vi "SetStringArray.vi"(4 "Sequence Context":refnum<k7>) -> (0 "error out":errorcluster)   [LabVIEW 2011]
doc: "Generates an array of string data and writes it to a TestStand Local Variable using the TestStand Utility VIs."
uses:
  <vilib>/addons/TestStand/_TSUtility.llb/TestStand - Set Property Value (String Array).vi
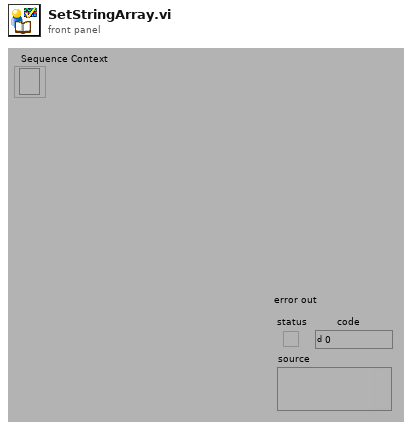
[diagram p1: front panel]
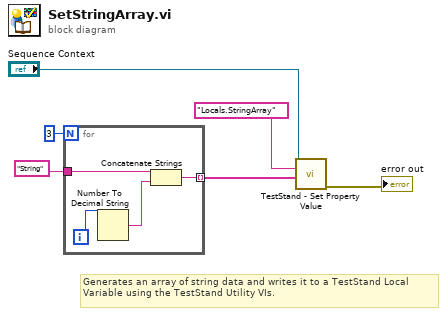
[diagram p0: block diagram]
diagram:
  # "Generates an array of string data and writes it to a TestStand Local Variable using the TestStand Utility VIs."
  n1 = for {
    N: 3 -> [_]
    tunnel: "String" -> [w9]
    tunnel: [w7] -> w3 mode=indexing
    i -> [w10]
    n2 = Number To Decimal String(number=w10) -> (decimal integer string=w8:string)  [unwired: 1 out]
    n3 = Concatenate Strings(w9, w8) -> (w7:string)
  }
  n4 = call-poly <vilib>:"TestStand - Set Property Value.vi"("Sequence Context In"="Sequence Context", "Lookup String"="Locals.StringArray", "New Value"=w3) -> ("error out"=→"error out":errorcluster)  [unwired: 2 in, 10 out]
